vi "Test Init Array.vi"() -> ()   [LabVIEW 2020]
panel:
  out "output array":dbl[](array[numeric])
  out "size(s)":i32
  out "initialized array":dbl[](array[numeric])
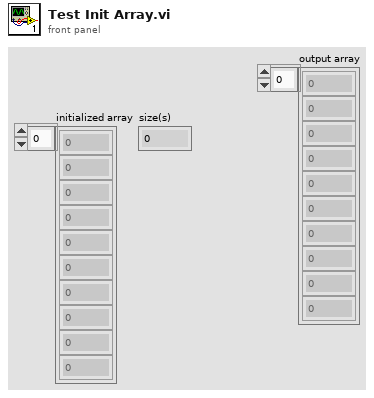
[diagram p1: front panel]
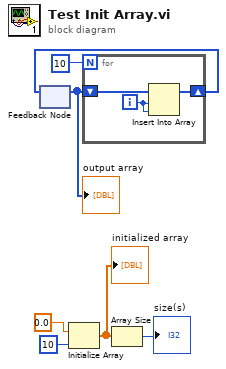
[diagram p0: block diagram]
diagram:
  n1 = feedback #1() -> (w1:i32[])  [unwired: 1 in]
  "output array" <- w1
  n2 = Initialize Array(0.0 ("element"), 10 ("dimension size")) -> (w4:dbl[])
  "initialized array" <- w4
  n3 = for {
    N: 10 -> [_]
    shift-right: [w9] -> w2
    shift-left: w1 -> [w8]
    i -> [w10]
    n4 = Insert Into Array(array=w8, index=w10, new element=w10) -> (w9:i32[])
  }
  n5 = feedback-in #1(w2) -> ()
  n6 = Array Size(array=w4) -> (size(s)=→"size(s)":i32)
